vi "DistortionCorrection.vi"(8 "error in (no error)":errorcluster, 10 "Grid Descriptor":cluster{"X Step":sgl, "Y Step":sgl, "Unit":T1}={"X Step"=5.0, "Y Step"=5.0, "Unit"=enum."Millimeter"}, 11 "File Path":path) -> (0 "error out":errorcluster, 3 "Corrected Image":T2(plugin-control))   [LabVIEW 2017]
uses:
  <vilib>/vision/Calibration.llb/Distortion Model.ctl
  <vilib>/vision/Calibration.llb/Distortion Model Types.ctl
  <vilib>/vision/NI_Vision_Development_Module.lvlib
panel:
  out "Original Image":T2(plugin-control)
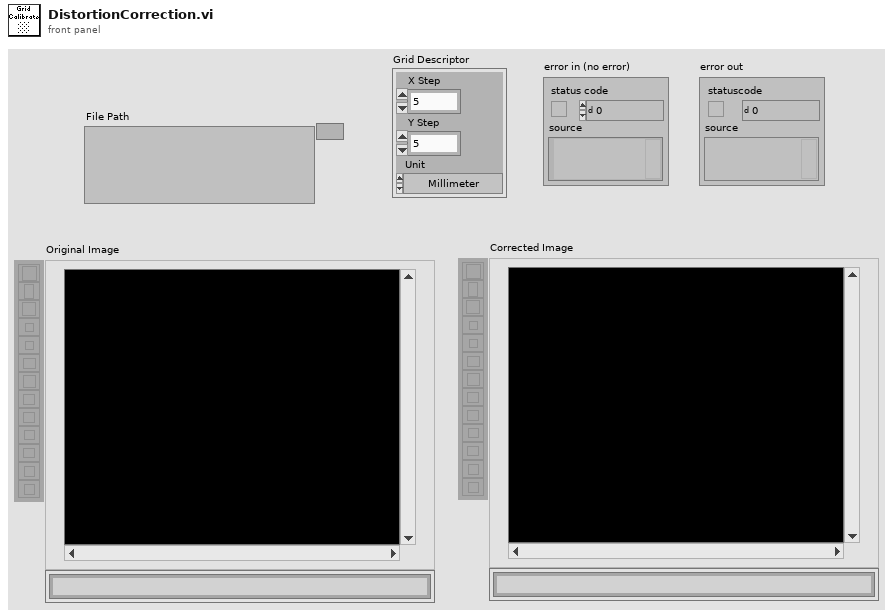
[diagram p1: front panel]
types:
  T1 = typedef "Image Unit" = enum32{"Undefined", "Angström", "Micrometer", "Millimeter", "Centimeter", "Meter", "Kilometer", "Microinch", "Inch", "Feet", "Nautical miles", "Standard miles", "Steps"}
  T2 = typedef "IMAQ Image.ctl" = refnum<image>
  T3 = typedef "Distortion Model.ctl" = cluster{"Distortion Model":T4, "Polynomial Model Setup":cluster{"Radial Coefficient":u32, "Tangential Coefficients ":bool}}
  T4 = typedef "Distortion Model Types.ctl" = i32
  T5 = typedef "Particle Parameters" = i32
  T6 = cluster{"Measurement Parameter":T5, "Range Lower Value":dbl, "Range Upper Value":dbl, "Range":bool, "Measurement Type":bool}[]
  T7 = typedef "Calibration Reference Points.ctl" = cluster{"Pixel Coordinates":cluster{"X":dbl, "Y":dbl}[], "Real World Coordinates":cluster{"X":dbl, "Y":dbl}[], "Unit":T1, "Image Size":cluster{"X":u32, "Y":u32}}
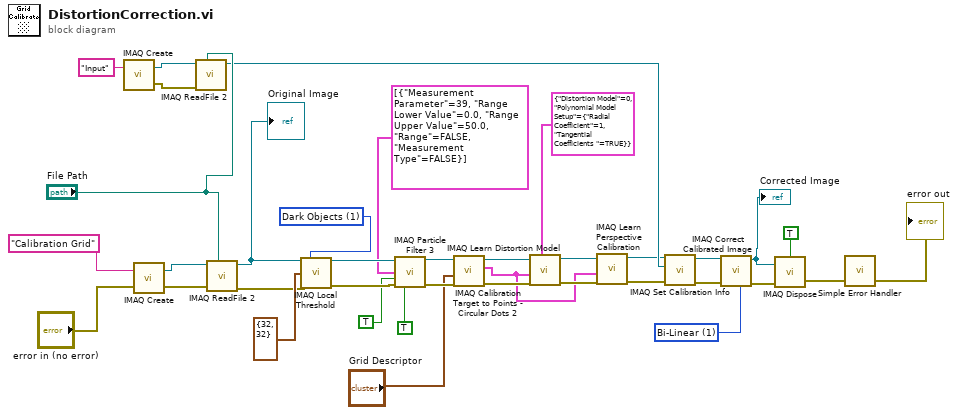
[diagram p0: block diagram]
diagram:
  w7 = u32 1 items=["Zero Order", "Bi-Linear", "Quadratic", "Cubic Spline"] ("Interpolation Type")
  w28 = u32 1 items=["Bright Objects", "Dark Objects"] ("Look For (Bright Objects)")
  n1 = call "IMAQ Create"("Image Name"="Input") -> ("New Image"=w34:T2, "error out"=w35:errorcluster)  [unwired: 4 in]
  n2 = call "IMAQ Create"("Image Name"="Calibration Grid", "error in (no error)"="error in (no error)") -> ("New Image"=w30:T2, "error out"=w29:errorcluster)  [unwired: 3 in]
  n3 = call "IMAQ ReadFile 2"("File Path"="File Path", "error in (no error)"=w35, "Image"=w34) -> ("Image Out"=w32:T2)  [unwired: 4 in, 4 out]
  n4 = call "IMAQ ReadFile 2"("File Path"="File Path", "error in (no error)"=w29, "Image"=w30) -> ("error out"=w26:errorcluster, "Image Out"=w3:T2)  [unwired: 4 in, 3 out]
  "Original Image" <- w3
  n5 = call "IMAQ Local Threshold"("Image Src"=w3, "Look For (Bright Objects)"=w28, "Window Size (32x32)"=cluster{"SizeX":i32, "SizeY":i32} {"SizeX"=32, "SizeY"=32}, "error in (no error)"=w26) -> ("Image Dst Out"=w21:T2, "error out"=w25:errorcluster)  [unwired: 10 in]
  n6 = call "IMAQ Particle Filter 3"("Image Src"=w21, "Selection Values"=T6 [{"Measurement Parameter"=39, "Range Lower Value"=0.0, "Range Upper Value"=50.0, "Range"=FALSE, "Measurement Type"=FALSE}], "Keep/Remove Particles (F)"=TRUE, "error in (no error)"=w25, "Reject Border? (F)"=TRUE) -> ("Image Dst Out"=w17:T2, "error out"=w24:errorcluster)  [unwired: 8 in, 1 out]
  n7 = call "IMAQ Calibration Target to Points - Circular Dots 2"("error in (no error)"=w24, "Grid Descriptor"="Grid Descriptor", "Target Image"=w17) -> ("error out"=w23:errorcluster, "Reference Points"=w15:T7, "Target Image (dup)"=w16:T2)  [unwired: 6 in]
  n8 = call "IMAQ Learn Distortion Model"("Distortion Model Setup"=T3 {"Distortion Model"=0, "Polynomial Model Setup"={"Radial Coefficient"=1, "Tangential Coefficients "=TRUE}}, "error in (no error)"=w23, "Reference Points"=w15, "Calibration Template Image"=w16) -> ("error out"=w22:errorcluster, "Calibration Template Image Out"=w14:T2)  [unwired: 6 in]
  n9 = call "IMAQ Learn Perspective Calibration"("error in (no error)"=w22, "Reference Points"=w15, "Calibration Template Image"=w14) -> ("error out"=w11:errorcluster, "Calibration Template Image Out"=w13:T2)  [unwired: 7 in]
  n10 = call "IMAQ Set Calibration Info"("error in (no error)"=w11, "Image Dst"=w32, "Image Src"=w13) -> ("error out"=w8:errorcluster, "Calibrated Image"=w10:T2)  [unwired: 7 in]
  n11 = call "IMAQ Correct Calibrated Image"("Interpolation Type"=w7, "error in (no error)"=w8, "Image Src"=w10) -> ("error out"=w5:errorcluster, "Corrected Image"=w9:T2)  [unwired: 7 in]
  "Corrected Image" <- w9
  n12 = call "IMAQ Dispose"("All Images? (No)"=TRUE, "Image"=w9, "error in (no error)"=w5) -> ("error out"=w4:errorcluster)  [unwired: 3 in]
  "error out" <- w4
  n13 = call <vilib>:"Simple Error Handler.vi"("error in (no error)"=w4) -> ()  [unwired: 4 in, 5 out]
